vi "SetLeftPaneSize.vi"(8 "error in (no error)":errorcluster, 9 "Left Pane Size":i32, 11 "Splitters":T1) -> (0 "error out":errorcluster)   [LabVIEW 2022 SP3, in "PentaPanesLibrary.lvlib" / "PentaPanes.lvclass"]
uses:
  PentaPanes.lvclass
  SplittersCluster.ctl
panel:
  out "In Range?":bool
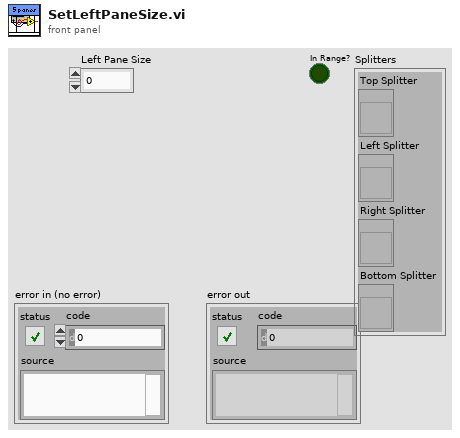
[diagram p1: front panel]
types:
  T1 = typedef "PentaPanesLibrary.lvlib/PentaPanes.lvclass/SplittersCluster.ctl" = cluster{"Top Splitter":refnum<vi>, "Left Splitter":refnum<vi>, "Right Splitter":refnum<vi>, "Bottom Splitter":refnum<vi>}
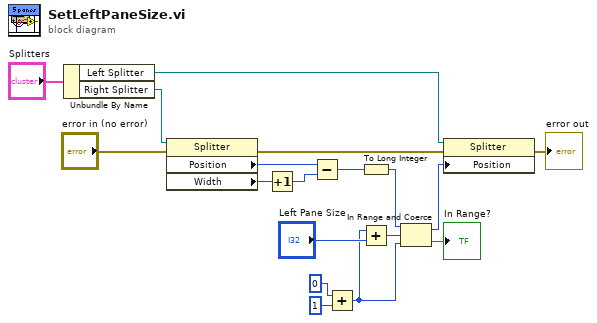
[diagram p0: block diagram]
diagram:
  n1 = Unbundle By Name("Splitters") -> ("Left Splitter"=w3:refnum<vi>, "Right Splitter"=w12:refnum<vi>)
  n2 = property class="Splitter"(reference=w12, error in="error in (no error)") -> (error out=w7:errorcluster, "Position"=w11:i32, "Width"=w5:u32)  [unwired: 1 out]
  n3 = Increment(x=w5) -> (x+1=w4:u32)
  n4 = Subtract(x=w11, y=w4) -> (x-y=w2:u32)
  n5 = Add(x=0, y=1 ("Splitter Position")) -> (x+y=w8:i32)
  n6 = To Long Integer(number=w2) -> (32bit integer=w1:i32)
  n7 = Add(x=w8, y="Left Pane Size") -> (x+y=w13:i32)
  n8 = In Range and Coerce(upper limit=w1, x=w13, lower limit=w8) -> (coerced(x)=w10:i32, In Range?=→"In Range?":bool)
  n9 = property class="Splitter"(reference=w3, error in=w7, "Position"=w10) -> (error out=→"error out":errorcluster)  [unwired: 1 out]
